vi "detection_camera.vi"() -> ()   [LabVIEW 2019]
uses:
  <vilib>/userDefined/High Color/IMAQdx.ctl
  <vilib>/vision/driver/IMAQdx.llb/IMAQdx Camera Control Mode.ctl
  <vilib>/vision/driver/NI_Vision_Acquisition_Software.lvlib
  <vilib>/vision/NI_Vision_Development_Module.lvlib
panel:
  in  "Settings":T1={"Algorithm"=2, "Number of Matches Requested"=1, "Minimum Match Score"=800.0, "SubPixel Accuracy"=TRUE, "Rotation Angle Ranges"=[], "Show Search Area"=FALSE, "Show Result"=TRUE} {"Rotation Angle Ranges"."End" format="%.1f"; "Rotation Angle Ranges"."Start" format="%.1f"; "Minimum Match Score" min=0 max=1000 format="%.2f"; "Number of Matches Requested" min=1; "Algorithm" items=["All", "Low Discrepancy Sampling", "Grayscale Value Pyramid", "Gradients Pyramid"]}
  in  "camera":T2="cam1"
  out "template":T3(plugin-control)
  out "Camera":T3(plugin-control)
  out "Out of NI Vision":T3(plugin-control)
  in  "File Path":path[](array[path])
  in  "Delay Time (s)":dbl(slide)=1.0 scale=0.0..10.0
  out "Number of Matches":i32
  out "Matches (pixel)":T4(array[cluster]) {"Bounding Box"."y" format="%.2f"; "Bounding Box"."x" format="%.2f"; "Position"."y" format="%.2f"; "Position"."x" format="%.2f"; "Score" format="%.2f"; "Scale" format="%.2f"; "Angle" format="%.2f"}
  in  "File Output Path":path
  in  "Image Quality":u32=750 max=1000 step=10
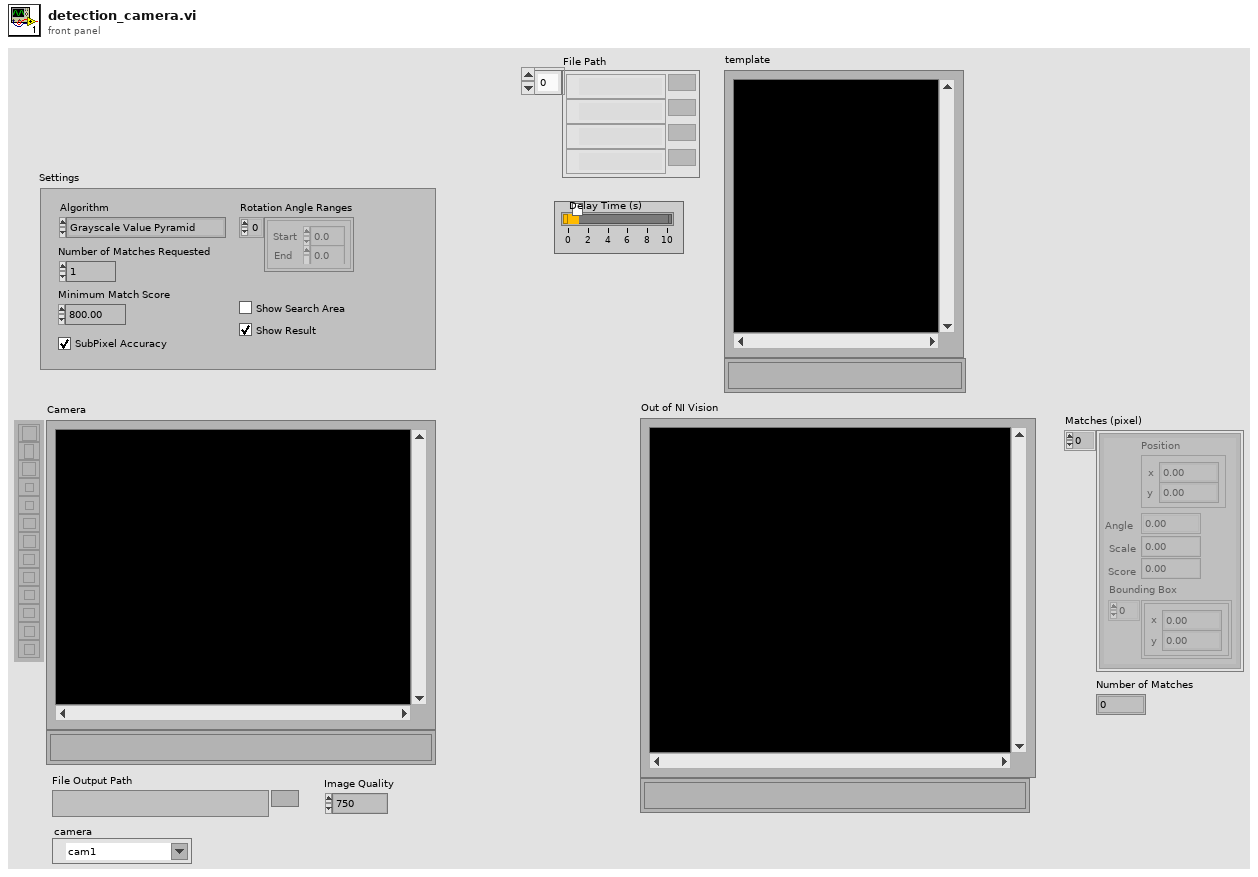
[diagram p1: front panel]
types:
  T1 = cluster{"Algorithm":i32, "Number of Matches Requested":i32, "Minimum Match Score":sgl, "SubPixel Accuracy":bool, "Rotation Angle Ranges":cluster{"Start":sgl, "End":sgl}[], "Show Search Area":bool, "Show Result":bool}
  T2 = typedef "IMAQdx.ctl" = refnum<k21>
  T3 = typedef "IMAQ Image.ctl" = refnum<image>
  T4 = cluster{"Position":cluster{"x":sgl, "y":sgl}, "Angle":sgl, "Scale":sgl, "Score":sgl, "Bounding Box":cluster{"x":sgl, "y":sgl}[]}[]
  T5 = typedef "NI_Vision_Acquisition_Software.lvlib/IMAQdx Camera Control Mode.ctl" = enum32{"Controller", "Listener"}
  T6 = cluster{"Rotation":bool, "Scale":bool, "Occlusion":bool, "Reserved":bool, "Reserved":bool, "Reserved":bool}
  T7 = typedef "Image Type" = u32
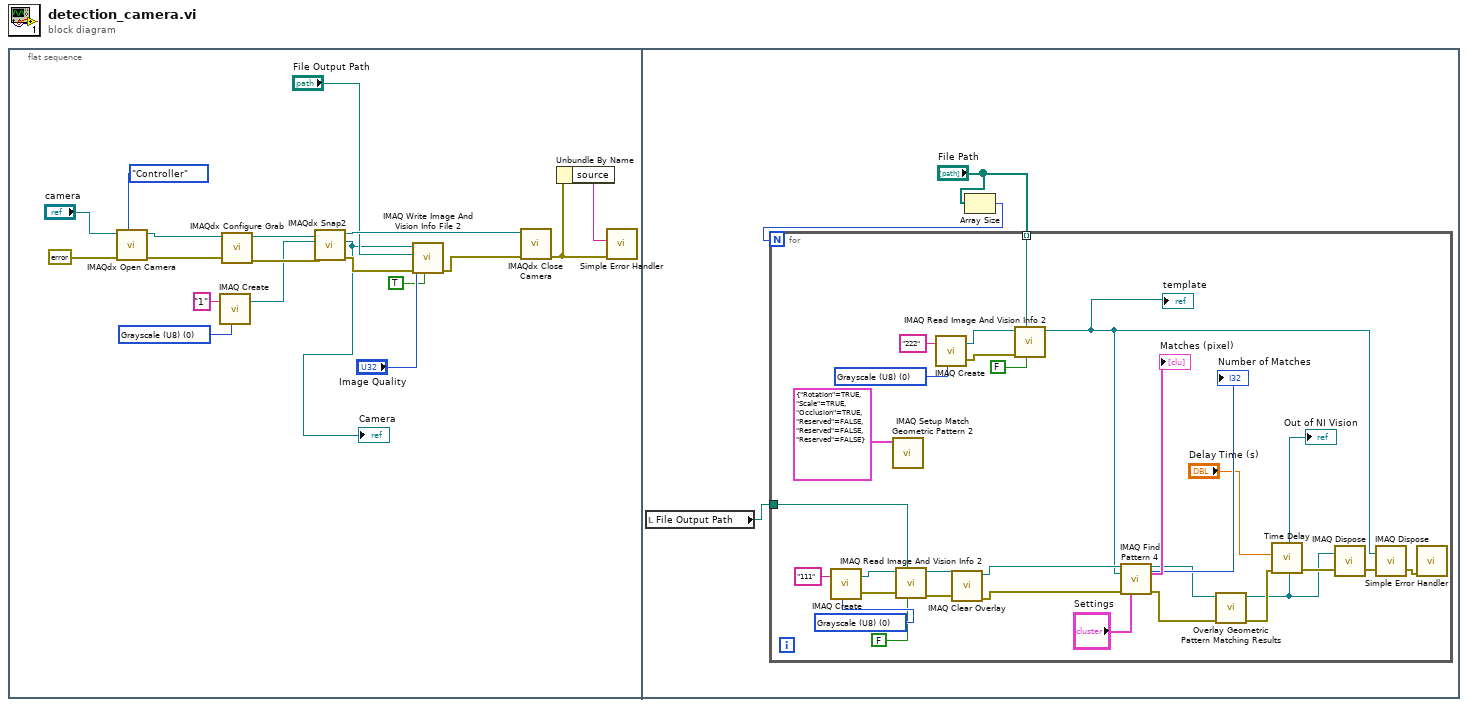
[diagram p0: block diagram]
diagram:
  n1 = flat-sequence {
    frame #0 {
      w15 = T7 0 items=["Grayscale (U8)", "Grayscale (I16)", "Grayscale (SGL)", "Complex (CSG)", "RGB (U32)", "HSL (U32)", "RGB (U64)", "Grayscale (U16)"] ("Image Type")
      n2 = call <vilib>:"IMAQdx Open Camera.vi"("Camera Control Mode"=IMAQdx_Camera_Control_Mode."Controller", "error in"=errorcluster {"status"=FALSE, "code"=0, "source"=""}, "Session In"="camera") -> ("error out"=w16:errorcluster, "Session Out"=w18:T2)  [unwired: 7 in]
      n3 = call "IMAQ Create"("Image Name"="1", "Image Type"=w15) -> ("New Image"=w7:T3)  [unwired: 3 in, 1 out]
      n4 = call <vilib>:"IMAQdx Configure Grab.vi"("error in"=w16, "Session In"=w18) -> ("error out"=w12:errorcluster, "Session Out"=w13:T2)  [unwired: 8 in]
      n5 = call <vilib>:"IMAQdx Snap2.vi"("error in"=w12, "Image In"=w7, "Session In"=w13) -> ("error out"=w10:errorcluster, "Image Out"=w2:T3, "Session Out"=w11:T2)  [unwired: 6 in]
      "Camera" <- w2
      n6 = call "IMAQ Write Image And Vision Info File 2"("Use bit depth? (false)"=TRUE, "error in (no error)"=w10, "Image Quality"="Image Quality", "File Path"="File Output Path", "Image"=w2) -> ("error out"=w9:errorcluster)  [unwired: 5 in, 1 out]
      n7 = call <vilib>:"IMAQdx Close Camera.vi"("error in"=w9, "Session In"=w11) -> ("error out"=w5:errorcluster)  [unwired: 9 in]
      n8 = Unbundle By Name(w5) -> ("source"=w4:string)
      n9 = call <vilib>:"Simple Error Handler.vi"("error source (\" \")"=w4, "error in (no error)"=w5) -> ()  [unwired: 3 in, 5 out]
    }
    frame #1 {
      n10 = local read "File Output Path"() -> (w22:path)
      n11 = Array Size(array="File Path") -> (size(s)=w20:i32)
      n12 = for {
        N: w20 -> [_]
        tunnel: w22 -> [w33]
        tunnel: "File Path" -> [w32] mode=indexing
        w44 = T7 0 items=["Grayscale (U8)", "Grayscale (I16)", "Grayscale (SGL)", "Complex (CSG)", "RGB (U32)", "HSL (U32)", "RGB (U64)", "Grayscale (U16)"] ("Image Type")
        w50 = T7 0 items=["Grayscale (U8)", "Grayscale (I16)", "Grayscale (SGL)", "Complex (CSG)", "RGB (U32)", "HSL (U32)", "RGB (U64)", "Grayscale (U16)"] ("Image Type")
        n13 = call "IMAQ Create"("Image Name"="111", "Image Type"=w50) -> ("New Image"=w47:T3, "error out"=w49:errorcluster)  [unwired: 3 in]
        n14 = call "IMAQ Setup Match Geometric Pattern 2"("Match Mode"=T6 {"Rotation"=TRUE, "Scale"=TRUE, "Occlusion"=TRUE, "Reserved"=FALSE, "Reserved"=FALSE, "Reserved"=FALSE}) -> ()  [unwired: 9 in, 2 out]
        n15 = call "IMAQ Read Image And Vision Info 2"("Use File Path Image Type"=FALSE, "File Path"=w33, "error in (no error)"=w49, "Image"=w47) -> ("error out"=w48:errorcluster, "Image Out"=w46:T3)  [unwired: 5 in, 1 out]
        n16 = call "IMAQ Create"("Image Name"="222", "Image Type"=w44) -> ("New Image"=w42:T3, "error out"=w43:errorcluster)  [unwired: 3 in]
        n17 = call "IMAQ Clear Overlay"("error in (no error)"=w48, "Image"=w46) -> ("error out"=w41:errorcluster, "Image Out"=w40:T3)  [unwired: 8 in]
        n18 = call "IMAQ Read Image And Vision Info 2"("Use File Path Image Type"=FALSE, "File Path"=w32, "error in (no error)"=w43, "Image"=w42) -> ("Image Out"=w26:T3)  [unwired: 5 in, 2 out]
        "template" <- w26
        n19 = call "IMAQ Find Pattern 4"("Image"=w40, "Template"=w26, "error in"=w41, "Settings"="Settings") -> ("Number of Matches"=→"Number of Matches":i32, "Image Out"=w29:T3, "Matches (pixel)"=→"Matches (pixel)":T4, "error out"=w30:errorcluster)  [unwired: 5 in, 3 out]
        n20 = call "Overlay Geometric Pattern Matching Results.vi"("error in"=w30, "Image"=w29) -> ("error out"=w28:errorcluster, "Image Out"=w27:T3)  [unwired: 8 in]
        "Out of NI Vision" <- w27
        n21 = call "Time Delay"("error in (no error)"=w28, "Delay Time (s)"="Delay Time (s)") -> ("error out"=w35:errorcluster)  [unwired: 9 in]
        n22 = call "IMAQ Dispose"("Image"=w27, "error in (no error)"=w35) -> ("error out"=w36:errorcluster)  [unwired: 4 in]
        n23 = call "IMAQ Dispose"("Image"=w26, "error in (no error)"=w36) -> ("error out"=w34:errorcluster)  [unwired: 4 in]
        n24 = call <vilib>:"Simple Error Handler.vi"("error in (no error)"=w34) -> ()  [unwired: 4 in, 5 out]
      }
    }
  }
